vi "DSF.Engine.Builder.Buffer.Parse.Process Transfer.vi"(6 "Data Type Buffers in in":T1, 8 "error in (no error)":errorcluster, 9 "VS Channel Buffer in":dbl[](array[numeric]), 10 "Transfer":refnum<class "DSF.Engine.Transfer.lvclass">, 11 "Builder in":refnum<class "DSF.Engine.Builder.lvclass">) -> (0 "error out":errorcluster, 1 "VS Channel Buffer out":dbl[](array[numeric]), 3 "Builder out":refnum<class "DSF.Engine.Builder.lvclass">, 4 "Data Type Buffers out":T1)   [LabVIEW 2016, in "DSF.Engine.lvlib" / "DSF.Engine.Builder.lvclass"]
uses:
  DSF.Engine.Builder.lvclass
  Typedefs/DSF.Engine.Typedefs.Type Buffers.ctl
  Transfer/DSF.Engine.Transfer.lvclass
  Transfer/DSF.Engine.Transfer.lvclass/DSF.Engine.Transfer.ctl
  Shared/Classes/Transfer/DSF.Shared.Configuration.Transfer.lvclass/DSF.Shared.Configuration.Transfer.ctl
  Buffer/DSF.Engine.Memory.Buffer.lvclass
  Shared/Classes/Transfer/DSF.Shared.Configuration.Transfer.lvclass
  Pointer/DSF.Engine.Pointer.VS Channels.lvclass
  DSF.Engine.lvlib
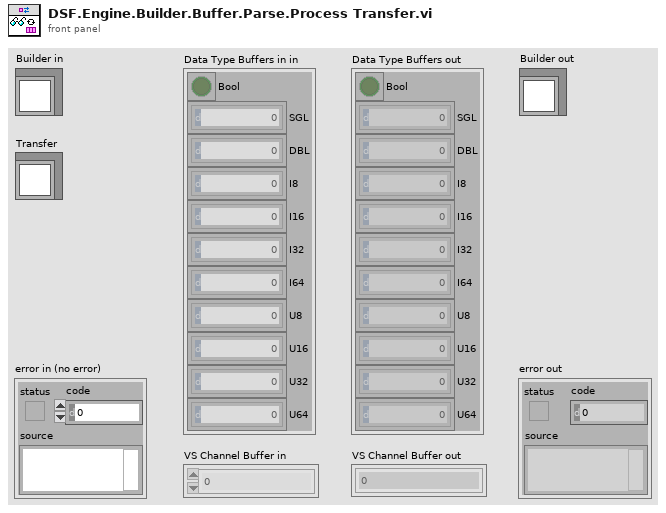
[diagram p1: front panel]
types:
  T1 = typedef "DSF.Engine.lvlib/DSF.Engine.Typedefs.Type Buffers.ctl" = cluster{"Bool":bool[], "SGL":sgl[], "DBL":dbl[], "I8":i8[], "I16":i16[], "I32":i32[], "I64":i64[], "U8":u8[], "U16":u16[], "U32":u32[], "U64":u64[]}
  T2 = typedef "DSF.Shared.lvlib/DSF.Shared.Typedefs.Configuration.Transfer.Channel Block Descriptor.ctl" = cluster{"First Channel Descriptor":T3, "count":u64, "vs channel index":u64}
  T3 = typedef "DSF.Shared.lvlib/DSF.Shared.Typedefs.Configuration.Transfer.Channel Descriptor.ctl" = cluster{"Channel Parameters":T4, "VS Channel Ref":T6}
  T4 = typedef "DSF.Shared.lvlib/DSF.Shared.Typedefs.Configuration.Transfer.Channel Parameters.ctl" = cluster{"offset":u64, "data type":T5}
  T5 = typedef "DSF.Shared.lvlib/DSF.Shared.Typedefs.Data Type.ctl" = enum8{"Bool", "SGL", "DBL", "I8", "I16", "I32", "I64", "U8", "U16", "U32", "U64"}
  T6 = typedef "Custom Device API.lvlib/Custom Device Item Ref.ctl" = u64
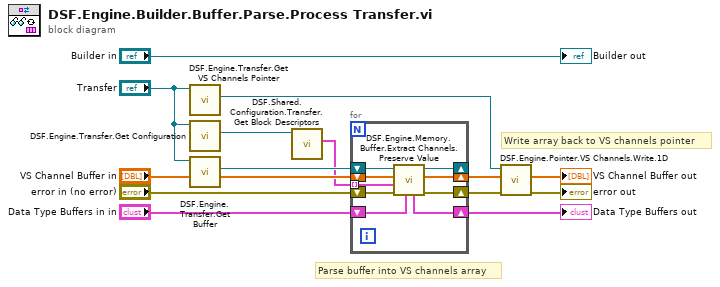
[diagram p0: block diagram]
diagram:
  # "Parse buffer into VS channels array"
  # "Write array back to VS channels pointer"
  n1 = call "DSF.Engine.Transfer.Get VS Channels Pointer.vi"("Transfer in"="Transfer") -> ("VS Channels Pointer"=w5:refnum<class "DSF.Engine.Pointer.VS Channels.lvclass">)  [unwired: 9 in, 1 out]
  n2 = call "DSF.Engine.Transfer.Get Configuration.vi"("Transfer in"="Transfer") -> ("Configuration"=w3:refnum<class "DSF.Shared.Configuration.Transfer.lvclass">)  [unwired: 9 in, 1 out]
  n3 = call "DSF.Engine.Transfer.Get Buffer.vi"("Transfer in"="Transfer") -> ("Buffer"=w4:refnum<class "DSF.Engine.Memory.Buffer.lvclass">)  [unwired: 9 in, 1 out]
  n4 = call "DSF.Shared.Configuration.Transfer.Get Block Descriptors.vi"("Transfer Configuration in"=w3) -> ("Channel Blocks"=w1:T2[])  [unwired: 8 in, 2 out]
  n5 = for {
    shift-right: [w21] -> w9
    shift-left: "VS Channel Buffer in" -> [w22]
    shift-right: [w20] -> w12
    shift-left: "error in (no error)" -> [w23]
    shift-right: [w17] -> w11
    shift-left: "Data Type Buffers in in" -> [w18]
    shift-right: [w16] -> _
    shift-left: w4 -> [w19]
    tunnel: w1 -> [w15] mode=indexing
    n6 = call "DSF.Engine.Memory.Buffer.Extract Channels.Preserve Value.vi"("Data Type Buffers in"=w18, "error in (no error)"=w23, "Channel Block"=w15, "VS Channels Array in"=w22, "Buffer in"=w19) -> ("error out"=w20:errorcluster, "VS Channels Array out"=w21:dbl[], "Buffer out"=w16:refnum<class "DSF.Engine.Memory.Buffer.lvclass">, "Data Type Buffers out"=w17:T1)  [unwired: 3 in]
  }
  "Data Type Buffers out" <- w11
  n7 = call "DSF.Engine.Pointer.VS Channels.Write.1D.vi"("error in (no error)"=w12, "Channels Array in"=w9, "VS Channels Pointer in"=w5) -> ("error out"=→"error out":errorcluster, "Channels Array out"=→"VS Channel Buffer out":dbl[])  [unwired: 5 in, 2 out]
  "Builder out" <- "Builder in"
